vi "dort_islem.vi"(8 "Ýþlem":string, 10 "Sayi2":string, 11 "Sayi1":string) -> (3 "Sonuç":dbl)   [LabVIEW 2019]
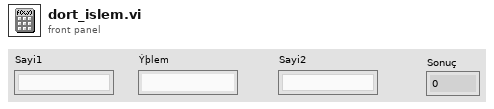
[diagram p1: front panel]
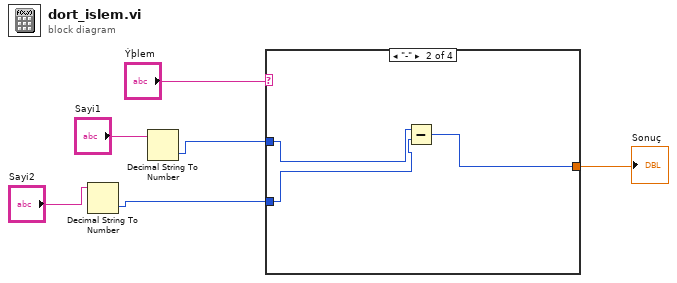
[diagram p0: block diagram]
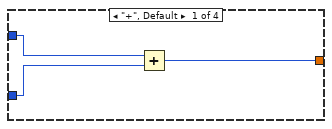
[diagram p2: hidden frame]
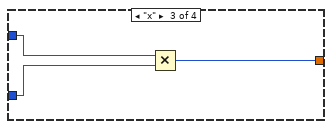
[diagram p3: hidden frame]
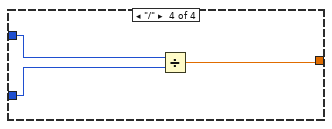
[diagram p4: hidden frame]
diagram:
  n1 = Decimal String To Number(string="Sayi2") -> (number=w4:i32)  [unwired: 2 in, 1 out]
  n2 = Decimal String To Number(string="Sayi1") -> (number=w1:i32)  [unwired: 2 in, 1 out]
  n3 = case shown="\"-\"" "Ýþlem" {
    tunnel: w1 -> [w9 w12 w15 w18]
    tunnel: w4 -> [w8 w11 w14 w17]
    tunnel: [w7 w10 w13 w16] -> w5
    frame "+", Default {
      n4 = Add(x=w9, y=w8) -> (x+y=w7:i32)
    }
    frame "-" {
      n5 = Subtract(x=w12, y=w11) -> (x-y=w10:i32)
    }
    frame "x" {
      n6 = Multiply(x=w15, y=w14) -> (x*y=w13:i32)
    }
    frame "/" {
      n7 = Divide(x=w18, y=w17) -> (x/y=w16:dbl)
    }
  }
  "Sonuç" <- w5
